vi "testBenchmarkSystemDefinitionFails.vi"(8 "error in (no error)":errorcluster, 11 "TestCase in":refnum<class "VeriStandTestCaseSystemTests.lvclass">) -> (0 "error out":errorcluster, 3 "TestCase out":refnum<class "VeriStandTestCaseSystemTests.lvclass">)   [LabVIEW 2017, in "VeriStandTestCaseSystemTests.lvclass"]
uses:
  VeriStandTestCaseSystemTests.lvclass
  VeriStandTestCase.lvclass
  <vilib>/addons/_JKI Toolkits/VI Tester/TestCase.llb/TestCase.lvclass
  C:/Program Files (x86)/National Instruments/LabVIEW 2017/vi.lib/addons/_JKI Toolkits/VI Tester/TestCase.llb/TestCase.lvclass
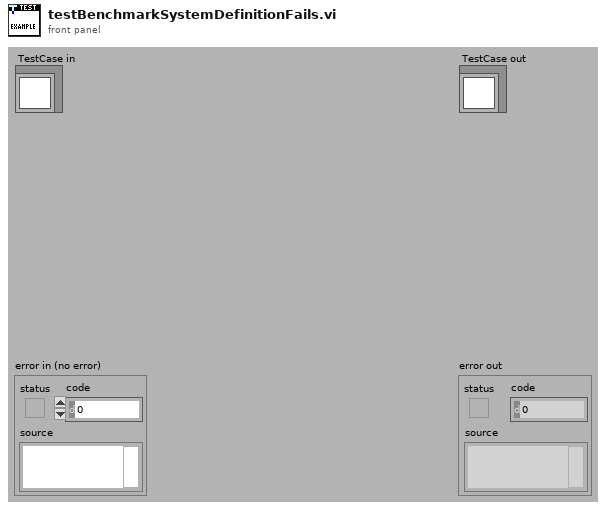
[diagram p1: front panel]
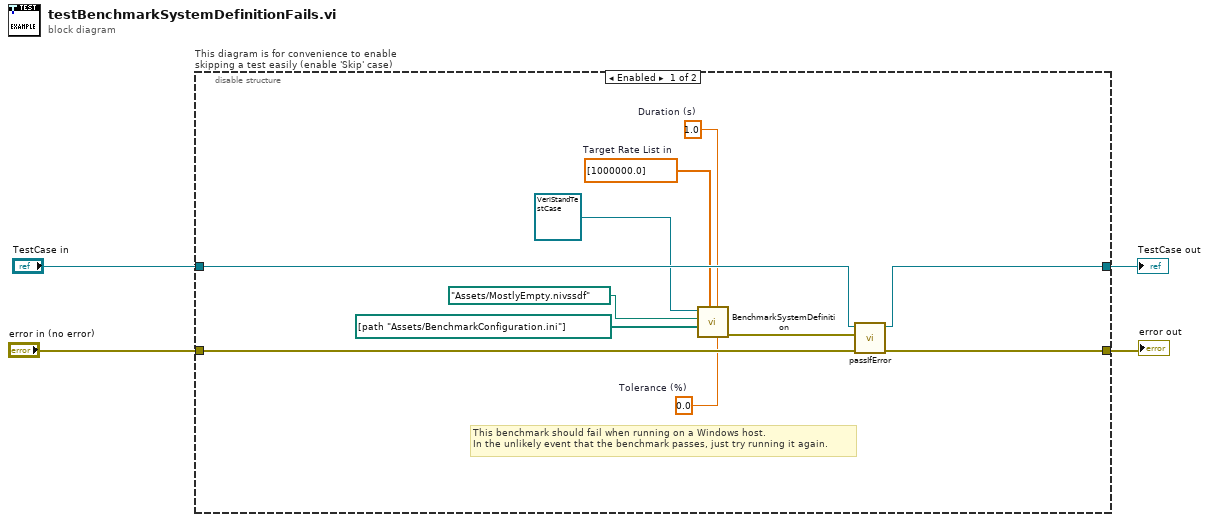
[diagram p0: block diagram]
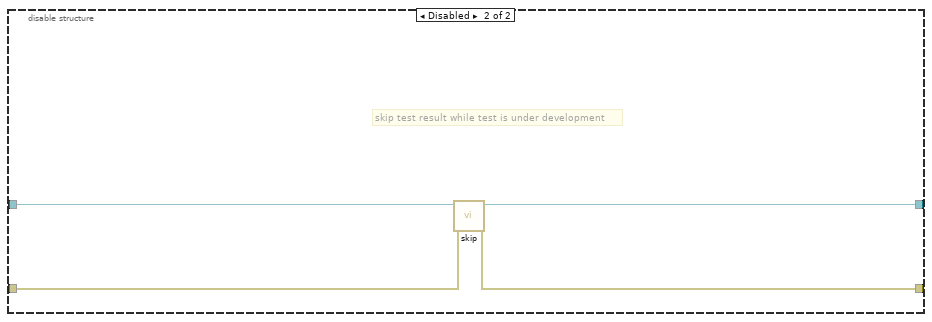
[diagram p2: hidden frame]
diagram:
  n1 = disable-structure "This diagram is for convenience to enable skipping a test easily (enable 'Skip' case)" shown="Enabled" {
    disable-tunnel: "TestCase in" -> [w13 w19]
    disable-tunnel: [w12 w17] -> w1
    disable-tunnel: [w14 w18] -> w3
    disable-tunnel: "error in (no error)" -> [w15 w16]
    frame Enabled {
      w6 = 0.0  # Tolerance (%)
      w7 = 1.0  # Duration (s)
      w8 = dbl[] [1000000.0]  # Target Rate List in
      # "This benchmark should fail when running on a Windows host.\nIn the unlikely event that the benchmark passes, just try running it again."
      n2 = call-dynamic "BenchmarkSystemDefinition.vi"("Tolerance (%)"=w6, "Duration (s)"=w7, "Target Rate List in"=w8, "overrides files"=path[] [path "Assets/BenchmarkConfiguration.ini"], "System Definition File"=path "Assets/MostlyEmpty.nivssdf", "VeriStandTestCase in"=refnum<class "VeriStandTestCase.lvclass"> refnum ("VeriStand Test Case in")) -> ("error out"=w11:errorcluster)  [unwired: 4 in, 1 out]
      n3 = call-dynamic "passIfError.vi"("error in (no error)"=w15, "error"=w11, "TestCase in"=w13) -> ("error out"=w14:errorcluster, "TestCase out"=w12:refnum<class "VeriStandTestCaseSystemTests.lvclass">)  [unwired: 7 in]
    }
    frame Disabled {
      # "skip test result while test is under development"
      n4 = call <vilib>:"skip.vi"("error in (no error)"=w16, "TestCase in"=w19) -> ("error out"=w18:errorcluster, "TestCase out"=w17:refnum<class "VeriStandTestCaseSystemTests.lvclass">)  [unwired: 8 in]
    }
  }
  "error out" <- w3
  "TestCase out" <- w1
